vi "String to Address.vi"(10 "Str":string) -> (2 "Type":u16, 3 "Address":i32[](array[numeric]))   [LabVIEW 2014]
panel:
  out "No":string[](array[string])
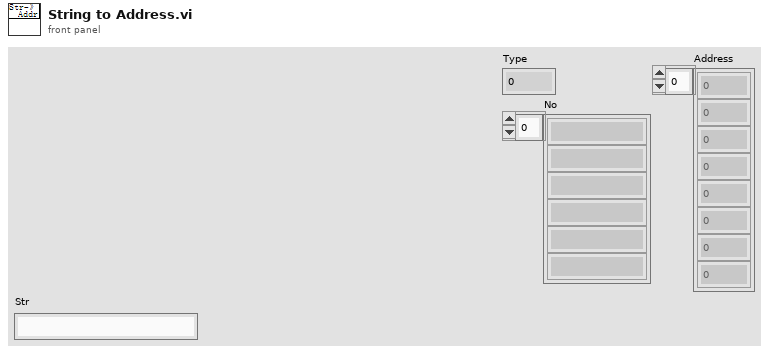
[diagram p1: front panel]
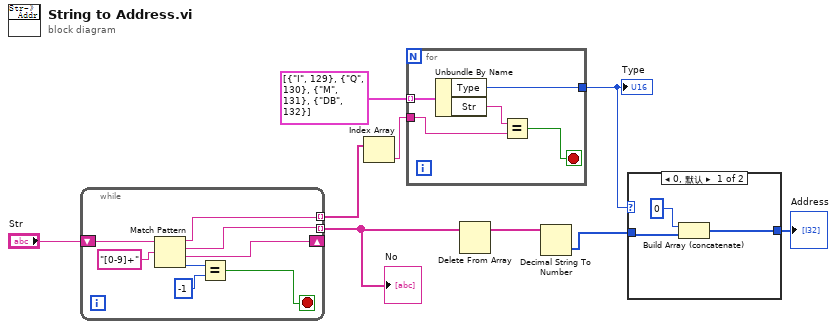
[diagram p0: block diagram]
diagram:
  n1 = while {
    shift-right: [w15] -> _
    shift-left: "Str" -> [w17]
    tunnel: [w14] -> w7 mode=indexing
    tunnel: [w13] -> w2 mode=indexing
    stop <- w10 stop-if-true
    n2 = Match Pattern(string=w17, regular expression="[0-9]+") -> (before substring=w14:string, match substring=w13:string, after substring=w15:string, offset past match=w12:i32)  [unwired: 1 in]
    n3 = Equal?(x=w12, y=-1) -> (x = y?=w10:bool)
  }
  "No" <- w2
  n4 = Index Array(array=w7) -> (element=w6:string)  [unwired: 1 in]
  n5 = for {
    tunnel: cluster{"Str":string, "Type":u16}[] [{"Str"="I", "Type"=129}, {"Str"="Q", "Type"=130}, {"Str"="M", "Type"=131}, {"Str"="DB", "Type"=132}] ("数组") -> [w22] mode=indexing
    tunnel: w6 -> [w20]
    tunnel: [w18] -> w5
    stop <- w19 stop-if-true
    n6 = Unbundle By Name(w22) -> ("Type"=w18:u16, "Str"=w21:string)
    n7 = Equal?(x=w21, y=w20) -> (x = y?=w19:bool)
  }
  "Type" <- w5
  n8 = Delete From Array(array=w2) -> (array with subset deleted=w1:string[])  [unwired: 2 in, 1 out]
  n9 = Decimal String To Number(string=w1) -> (number=w3:i32[])  [unwired: 2 in, 1 out]
  n10 = case shown="0, 默认" w5 {
    tunnel: w3 -> [w25 w26]
    tunnel: [w24 w26] -> w4
    frame 0, Default {
      n11 = Build Array (concatenate)(0, w25) -> (w24:i32[])
    }
    frame 132 {
    }
  }
  "Address" <- w4
